vi "to_V.vi"(8 "Gain":i32=10, 11 "DataBuffer":u16[](array[numeric])) -> (3 "value":dbl[](array[numeric]))   [LabVIEW 2012]
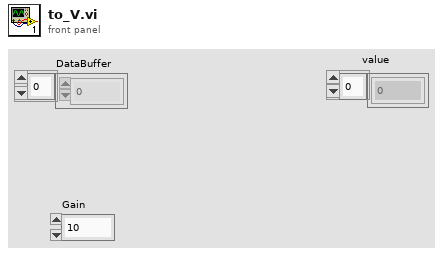
[diagram p1: front panel]
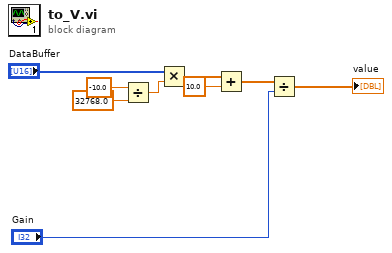
[diagram p0: block diagram]
diagram:
  n1 = Divide(x=-10.0, y=32768.0) -> (x/y=w7:dbl)
  n2 = Multiply(x="DataBuffer", y=w7) -> (x*y=w6:dbl[])
  n3 = Add(x=w6, y=10.0) -> (x+y=w3:dbl[])
  n4 = Divide(x=w3, y="Gain") -> (x/y=→"value":dbl[])
